vi "SVGlobal_ReadStat.vi"() -> ()   [LabVIEW 2020, in "Shared Variable Interface.lvlib"]
uses:
  Shared Variable Interface.lvlib
panel:
  in  "ReadRate":dbl
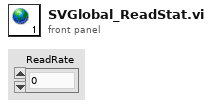
[diagram p1: front panel]
diagram:
